vi "PROCESS_COUNTER_SIGNALS.vi"(11 "Signal Array In":dynamicdata[](array[waveform])) -> (3 "Signal Array Out":dynamicdata[](array[waveform]))   [LabVIEW 2013]
uses:
  <vilib>/express/express shared/transition.llb/Dynamic To Waveform Array.vi
  <vilib>/express/express signal manip/GetorSetDDTAttributes/Set DDT Attributes/SetT0.vi
  <vilib>/express/express shared/transition.llb/Waveform Array To Dynamic.vi
  <vilib>/express/express signal manip/GetorSetDDTAttributes/Set DDT Attributes/Set DDT Properties.xnode
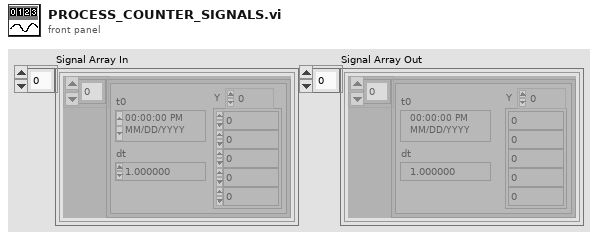
[diagram p1: front panel]
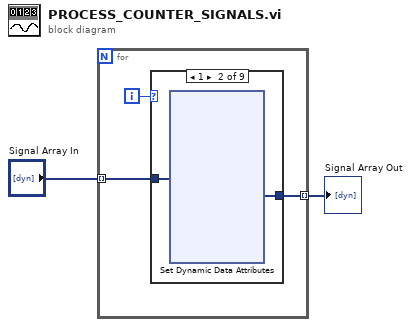
[diagram p0: block diagram]
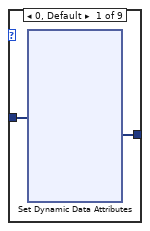
[diagram p2: hidden frame]
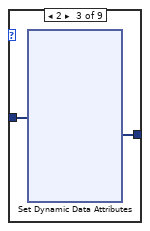
[diagram p3: hidden frame]
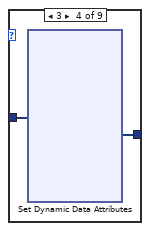
[diagram p4: hidden frame]
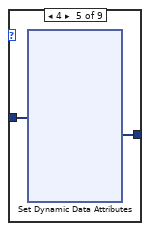
[diagram p5: hidden frame]
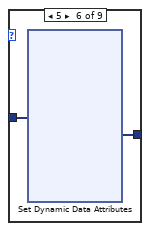
[diagram p6: hidden frame]
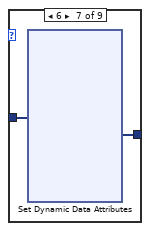
[diagram p7: hidden frame]
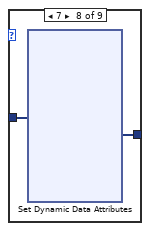
[diagram p8: hidden frame]
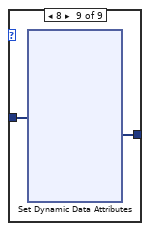
[diagram p9: hidden frame]
diagram:
  n1 = for {
    tunnel: [w4] -> w2 mode=indexing
    tunnel: "Signal Array In" -> [w3] mode=indexing
    i -> [w5]
    n2 = case shown="1" w5 {
      tunnel: w3 -> [w7 w26 w47 w67 w87 w107 w126 w147 w167]
      tunnel: [w6 w27 w46 w66 w86 w106 w127 w146 w166] -> w4
      frame 0, Default {
        n3 = xnode "Set Dynamic Data Attributes"("Signals In"=w7) -> ("Signals Out"=w6:dynamicdata)  [unwired: 4 in, 1 out]
      }
      frame 1 {
        n4 = xnode "Set Dynamic Data Attributes"("Signals In"=w26) -> ("Signals Out"=w27:dynamicdata)  [unwired: 4 in, 1 out]
      }
      frame 2 {
        n5 = xnode "Set Dynamic Data Attributes"("Signals In"=w47) -> ("Signals Out"=w46:dynamicdata)  [unwired: 4 in, 1 out]
      }
      frame 3 {
        n6 = xnode "Set Dynamic Data Attributes"("Signals In"=w67) -> ("Signals Out"=w66:dynamicdata)  [unwired: 4 in, 1 out]
      }
      frame 4 {
        n7 = xnode "Set Dynamic Data Attributes"("Signals In"=w87) -> ("Signals Out"=w86:dynamicdata)  [unwired: 4 in, 1 out]
      }
      frame 5 {
        n8 = xnode "Set Dynamic Data Attributes"("Signals In"=w107) -> ("Signals Out"=w106:dynamicdata)  [unwired: 4 in, 1 out]
      }
      frame 6 {
        n9 = xnode "Set Dynamic Data Attributes"("Signals In"=w126) -> ("Signals Out"=w127:dynamicdata)  [unwired: 4 in, 1 out]
      }
      frame 7 {
        n10 = xnode "Set Dynamic Data Attributes"("Signals In"=w147) -> ("Signals Out"=w146:dynamicdata)  [unwired: 4 in, 1 out]
      }
      frame 8 {
        n11 = xnode "Set Dynamic Data Attributes"("Signals In"=w167) -> ("Signals Out"=w166:dynamicdata)  [unwired: 4 in, 1 out]
      }
    }
  }
  "Signal Array Out" <- w2
